vi "Open Instrument.vi"(8 "error in (no error)":errorcluster, 11 "instrument.PPMS2 in":refnum<class "instrument.PPMS.lvclass">) -> (0 "error out":errorcluster, 3 "instrument.PPMS2 out":refnum<class "instrument.PPMS.lvclass">)   [LabVIEW 2016, in "instrument.PPMS.lvclass"]
uses:
  instrument.PPMS.lvclass
  instrument.PPMS.lvclass/instrument.PPMS.ctl
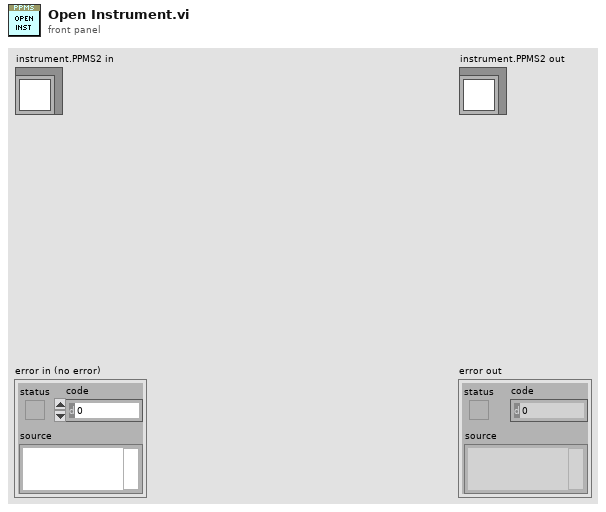
[diagram p1: front panel]
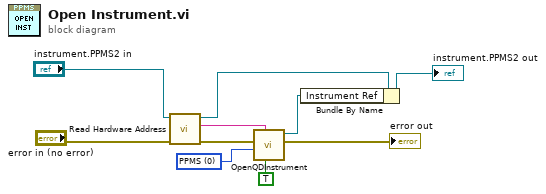
[diagram p0: block diagram]
diagram:
  w9 = 0 items=["PPMS", "VersaLab", "DynaCool", "SVSM"] ("Instrument\nType")
  n1 = call-dynamic "Read Hardware Address.vi"("error in (no error)"="error in (no error)", "Instrument in"="instrument.PPMS2 in") -> ("error out"=w6:errorcluster, "Hardware Address"=w5:string, "Instrument out"=w3:refnum<class "instrument.PPMS.lvclass">)  [unwired: 7 in]
  n2 = call "OpenQDInstrument.vi"("Remote"=TRUE, "IP Address"=w5, "Instrument Type"=w9, "error in (no error)"=w6) -> ("error out"=→"error out":errorcluster, "Instrument Ref"=w1:refnum<k24>)  [unwired: 4 in]
  n3 = Bundle By Name(cluster=w3, "Instrument Ref"=w1) -> (→"instrument.PPMS2 out":refnum<class "instrument.PPMS.lvclass">)
